vi "Read Single Value.vi"(8 "error in (no error)":errorcluster, 10 "Channel":refnum<k21>, 11 "DAQmx in":refnum<class "DAQmx.lvclass">) -> (0 "error out":errorcluster, 2 "Value":dbl format="%0.2f", 3 "DAQmx out":refnum<class "DAQmx.lvclass">)   [LabVIEW 2015, in "DAQmx.lvclass"]
uses:
  DAQmx.lvclass
  <vilib>/DAQmx/read.llb/DAQmx Read (Analog DBL 1Chan 1Samp).vi
  <vilib>/DAQmx/miscellaneous.llb/DAQmx Fill In Error Info.vi
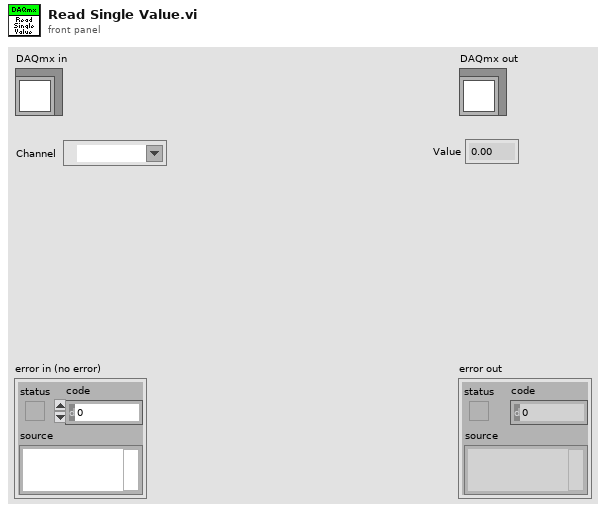
[diagram p1: front panel]
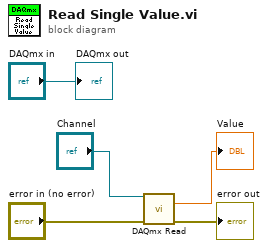
[diagram p0: block diagram]
diagram:
  n1 = call-poly <vilib>:"DAQmx Read.vi"("task/channels in"="Channel", "error in"="error in (no error)") -> ("data"=→"Value":dbl, "error out"=→"error out":errorcluster)  [unwired: 11 in, 1 out]
  "DAQmx out" <- "DAQmx in"
